vi "init.vi"(8 "error in (no error)":errorcluster, 10 "Variant":variant, 11 "PSP-603 in":refnum<class "PSP-603.lvclass">) -> (0 "error out":errorcluster, 3 "PSP-603 out":refnum<class "PSP-603.lvclass">)   [LabVIEW 2025, in "Power Supply.lvlib" / "PSP-603.lvclass"]
uses:
  PSP-603.lvclass
  PSP-603.lvclass/PSP-603.ctl
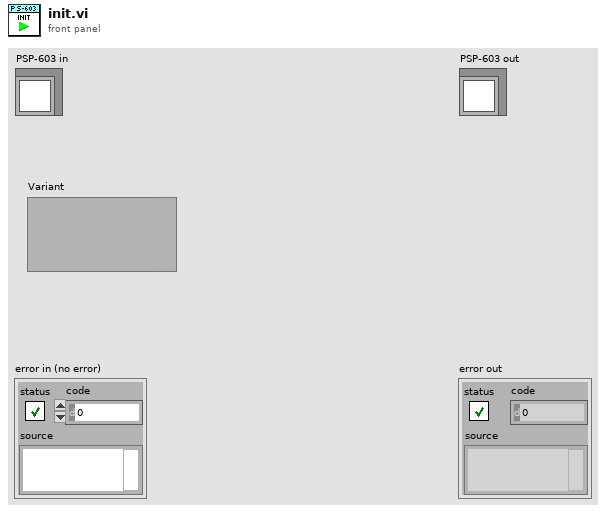
[diagram p1: front panel]
types:
  T1 = cluster{"Baud_Rate":u16, "Data_Bits":u16, "Parity":u16, "Stop_Bits":u16, "Flow_Control":u16, "Termination_Char":u8, "Receive Termination Char?":bool, "Send Termination Char?":bool}
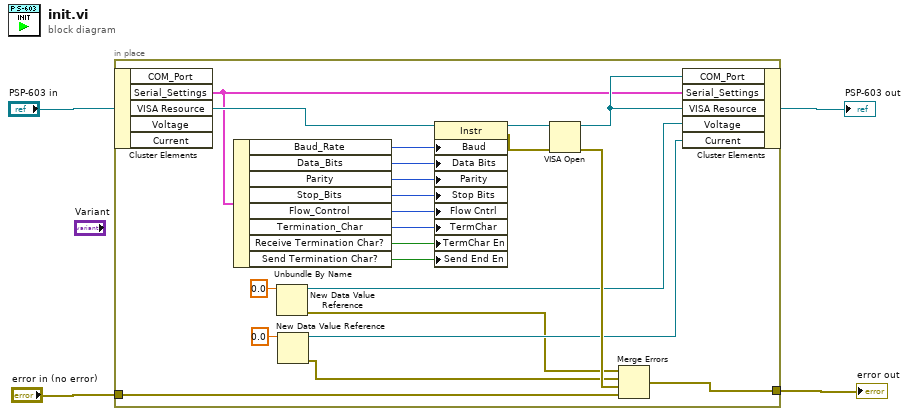
[diagram p0: block diagram]
diagram:
  n1 = in-place {
    in-place-border: [w11] -> w2
    in-place-border: "error in (no error)" -> [w12]
    n2 = in-place-cluster #1("PSP-603 in") -> ("Serial_Settings"=w14:T1, "VISA Resource"=w26:refnum<visa-resource-name>)  [unwired: 3 out]
    n3 = Unbundle By Name(w14) -> ("Baud_Rate"=w25:u16, "Data_Bits"=w24:u16, "Parity"=w23:u16, "Stop_Bits"=w22:u16, "Flow_Control"=w21:u16, "Termination_Char"=w20:u8, "Receive Termination Char?"=w19:bool, "Send Termination Char?"=w18:bool)
    n4 = New Data Value Reference(data value=0.0) -> (data value reference=w8:refnum<data-value>, error out=w5:errorcluster)  [unwired: 1 in]
    n5 = New Data Value Reference(data value=0.0) -> (data value reference=w7:refnum<data-value>, error out=w6:errorcluster)  [unwired: 1 in]
    n6 = property class="Instr"(reference=w26, "Baud"=w25, "Data Bits"=w24, "Parity"=w23, "Stop Bits"=w22, "Flow Cntrl"=w21, "TermChar"=w20, "TermChar En"=w19, "Send End En"=w18) -> (reference out=w17:refnum<visa-resource-name>, error out=w16:errorcluster)  [unwired: 1 in]
    n7 = VISA Open(error in (no error)=w16, VISA resource name=w17) -> (VISA resource name=w15:refnum<visa-resource-name>, error out=w13:errorcluster)  [unwired: 3 in]
    n8 = Merge Errors(w5, w6, w13, w12) -> (w11:errorcluster)
    n9 = in-place-cluster #1("COM_Port"=w15, "Serial_Settings"=w14, "VISA Resource"=w15, "Voltage"=w8, "Current"=w7) -> (→"PSP-603 out":refnum<class "PSP-603.lvclass">)
  }
  "error out" <- w2
